vi "ROI坐标转换2.vi"() -> ()   [LabVIEW 2018]
uses:
  <vilib>/vision/NI_Vision_Development_Module.lvlib
panel:
  out "Image":T1(plugin-control)
  in  "路径":path
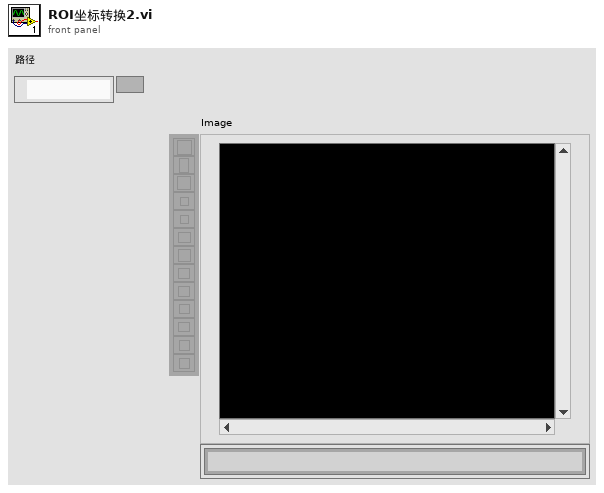
[diagram p1: front panel]
types:
  T1 = typedef "IMAQ Image.ctl" = refnum<image>
  T2 = cluster{"Origin":cluster{"X":sgl, "Y":sgl}, "Angle (deg)":sgl, "Axis Reference":u32}
  T3 = typedef "IMAQ Rectangle" = cluster{"Left":i32, "Top":i32, "Right":i32, "Bottom":i32, "Rotation":dbl}
  T4 = typedef "ROI Descriptor" = cluster{"Global Rectangle":i32[], "Contours":cluster{"ID":enum32{"External", "Internal"}, "Type":u32, "Coordinates":i32[]}[]}
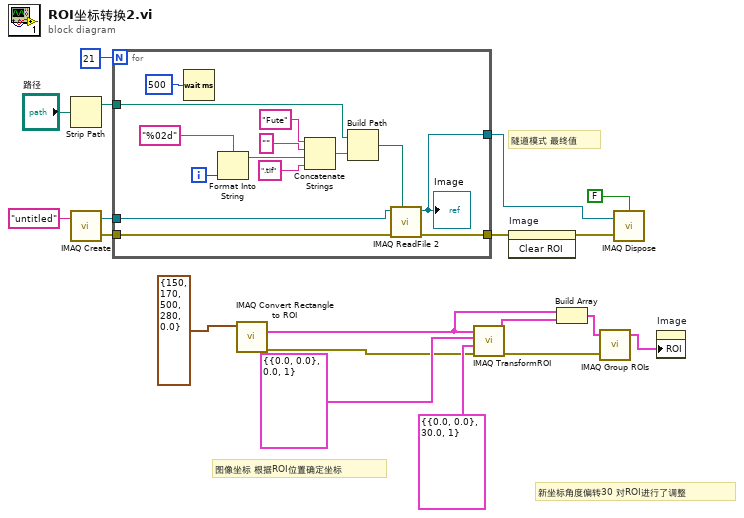
[diagram p0: block diagram]
diagram:
  # "新坐标角度偏转30 对ROI进行了调整"
  # "图像坐标 根据ROI位置确定坐标"
  # "隧道模式 最终值"
  n1 = Strip Path(path="路径") -> (stripped path=w17:path)  [unwired: 1 out]
  n2 = call "IMAQ Create"("Image Name"="untitled") -> ("New Image"=w16:T1, "error out"=w15:errorcluster)  [unwired: 4 in]
  n3 = for {
    N: 21 -> [_]
    tunnel: w17 -> [w24]
    tunnel: w16 -> [w33]
    tunnel: w15 -> [w32]
    tunnel: [w22] -> w13
    tunnel: [w21] -> w11
    i -> [w31]
    n4 = Wait (ms)(milliseconds to wait=u32 500 ("等待时间（毫秒）")) -> ()  [unwired: 1 out]
    n5 = Format Into String(format string="%02d" ("格式字符串"), w31) -> (resulting string=w29:string)  [unwired: 2 in, 1 out]
    n6 = Concatenate Strings("Fute" ("字符串"), "" ("字符串"), w29, ".tif" ("字符串")) -> (w25:string)
    n7 = Build Path(base path=w24, name or relative path=w25) -> (appended path=w23:path)
    n8 = call "IMAQ ReadFile 2"("File Path"=w23, "error in (no error)"=w32, "Image"=w33) -> ("error out"=w22:errorcluster, "Image Out"=w21:T1)  [unwired: 4 in, 3 out]
    "Image" <- w21
  }
  n9 = call "IMAQ Convert Rectangle to ROI"("Rectangle"=T3 {"Left"=150, "Top"=170, "Right"=500, "Bottom"=280, "Rotation"=0.0}) -> ("error out"=w3:errorcluster, "ROI Descriptor"=w6:T4)  [unwired: 8 in]
  n10 = call "IMAQ TransformROI"("error in (no error)"=w3, "New Reference"=T2 {"Origin"={"X"=0.0, "Y"=0.0}, "Angle (deg)"=30.0, "Axis Reference"=1}, "Base Reference"=T2 {"Origin"={"X"=0.0, "Y"=0.0}, "Angle (deg)"=0.0, "Axis Reference"=1}, "ROI Descriptor"=w6) -> ("error out"=w2:errorcluster, "ROI Descriptor out"=w5:T4)  [unwired: 6 in]
  n11 = invoke on="Image" class="ImageControl" method="Clear ROI"(error in=w13) -> (error out=w12:errorcluster)  [unwired: 2 in, 2 out]
  n12 = Build Array(w6, w5) -> (w4:T4[])
  n13 = call "IMAQ Group ROIs"("error in (no error)"=w2, "ROI Descriptors"=w4) -> ("ROI Descriptor out"=w1:T4)  [unwired: 2 in, 1 out]
  n14 = call "IMAQ Dispose"("All Images? (No)"=FALSE, "Image"=w11, "error in (no error)"=w12) -> ()  [unwired: 3 in, 1 out]
  n15 = property on="Image" class="ImageControl"("ROI"=w1) -> ()  [unwired: 2 in, 2 out]
